vi "Read Header Text.vi"(8 "error in (no error)":errorcluster, 11 "Set Header Text in":refnum<class "Set Header Text.lvclass">) -> (0 "error out":errorcluster, 2 "Header Text":string, 3 "Set Header Text out":refnum<class "Set Header Text.lvclass">)   [LabVIEW 2011, in "Set Header Text.lvclass"]
uses:
  Set Header Text.lvclass
  Set Header Text.lvclass/Set Header Text.ctl
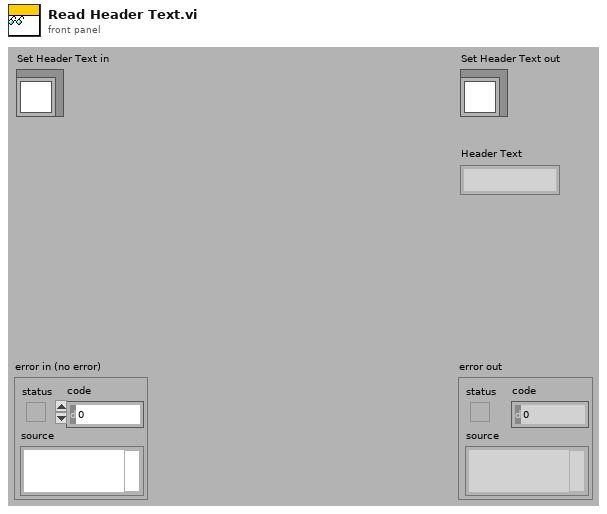
[diagram p1: front panel]
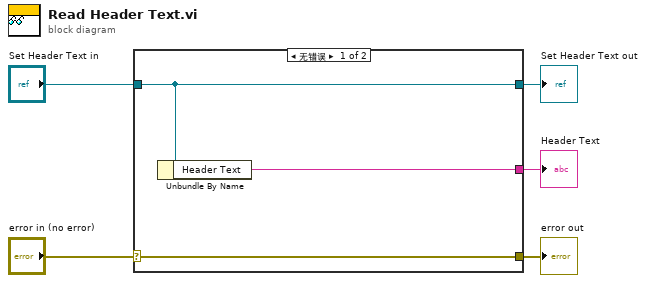
[diagram p0: block diagram]
diagram:
  n1 = case shown="无错误" "error in (no error)" {
    selector: "error in (no error)" -> [w8 w9]
    tunnel: [w8 w9] -> w4
    tunnel: [w7 w10] -> w2
    tunnel: "Set Header Text in" -> [w7 w10]
    tunnel: [w6 _] -> w1
    frame No Error {
      n2 = Unbundle By Name(w7) -> ("Header Text"=w6:string)
    }
    frame Error {
    }
  }
  "error out" <- w4
  "Set Header Text out" <- w2
  "Header Text" <- w1
